vi "Spaceship_Draw.vi"(1 "Spaceship_data out":T1) -> (0 "SpaceshipLines":cluster{"x":i16, "y":i16}[](array[cluster]))   [LabVIEW 2017]
uses:
  Spaceship_data.ctl
  GameConfig/GameConfig_data.ctl
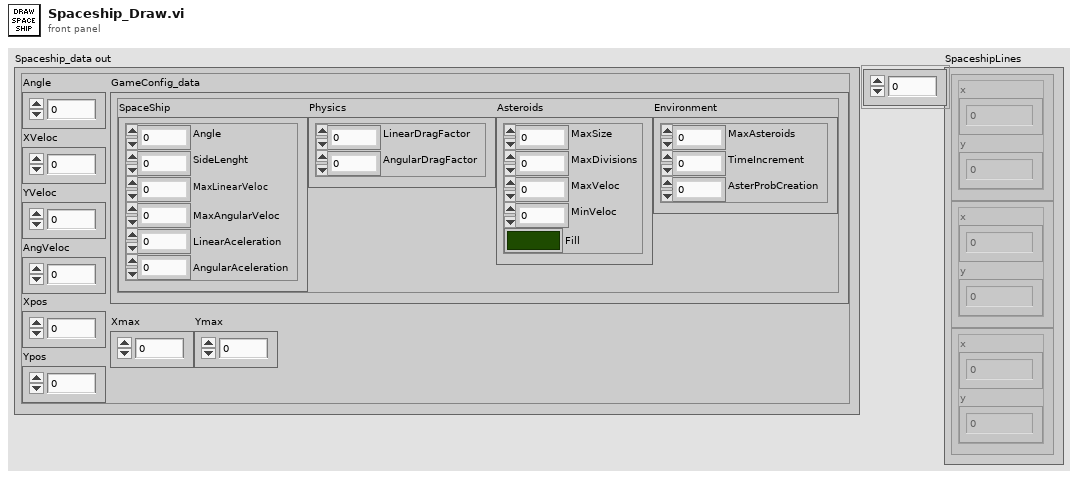
[diagram p1: front panel]
types:
  T1 = typedef "Spaceship_data.ctl" = cluster{"Angle":dbl, "XVeloc":dbl, "YVeloc":dbl, "AngVeloc":dbl, "GameConfig_data":T2, "Xpos":dbl, "Ypos":dbl, "Xmax":dbl, "Ymax":dbl}
  T2 = typedef "GameConfig_data.ctl" = cluster{"SpaceShip":cluster{"Angle":dbl, "SideLenght":dbl, "MaxLinearVeloc":dbl, "MaxAngularVeloc":dbl, "LinearAceleration":dbl, "AngularAceleration":dbl}, "Physics":cluster{"LinearDragFactor":dbl, "AngularDragFactor":dbl}, "Asteroids":cluster{"MaxSize":dbl, "MaxDivisions":i32, "MaxVeloc":dbl, "MinVeloc":dbl, "Fill":bool}, "Environment":cluster{"MaxAsteroids":i32, "TimeIncrement":dbl, "AsterProbCreation":dbl}}
  T3 = cluster{"Angle":dbl, "SideLenght":dbl, "MaxLinearVeloc":dbl, "MaxAngularVeloc":dbl, "LinearAceleration":dbl, "AngularAceleration":dbl}
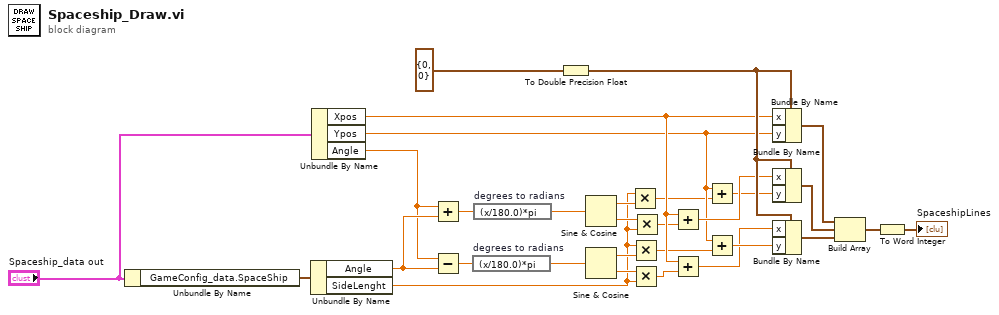
[diagram p0: block diagram]
diagram:
  n1 = Unbundle By Name("Spaceship_data out") -> ("GameConfig_data.SpaceShip"=w28:T3)
  n2 = Unbundle By Name(w28) -> ("Angle"=w27:dbl, "SideLenght"=w3:dbl)
  n3 = Unbundle By Name("Spaceship_data out") -> ("Xpos"=w20:dbl, "Ypos"=w19:dbl, "Angle"=w26:dbl)
  n4 = Add(x=w26, y=w27) -> (x+y=w11:dbl)
  n5 = Subtract(x=w26, y=w27) -> (x-y=w13:dbl)
  n6 = expression code="(x/180.0)*pi" "degrees to radians"(w13) -> (w12:dbl)
  n7 = expression code="(x/180.0)*pi" "degrees to radians"(w11) -> (w10:dbl)
  n8 = To Double Precision Float(number=cluster{"x":i16, "y":i16} {"x"=0, "y"=0}) -> (double precision float=w30:cluster{"x":dbl, "y":dbl})
  n9 = Sine & Cosine(0:w10) -> (1:w5:dbl, 2:w4:dbl)
  n10 = Sine & Cosine(0:w12) -> (1:w7:dbl, 2:w9:dbl)
  n11 = Multiply(x=w3, y=w5) -> (x*y=w1:dbl)
  n12 = Multiply(x=w3, y=w7) -> (x*y=w6:dbl)
  n13 = Multiply(x=w9, y=w3) -> (x*y=w8:dbl)
  n14 = Multiply(x=w4, y=w3) -> (x*y=w2:dbl)
  n15 = Add(x=w20, y=w2) -> (x+y=w24:dbl)
  n16 = Add(x=w20, y=w8) -> (x+y=w21:dbl)
  n17 = Add(x=w19, y=w1) -> (x+y=w23:dbl)
  n18 = Add(x=w19, y=w6) -> (x+y=w22:dbl)
  n19 = Bundle By Name(cluster=w30, "x"=w20, "y"=w19) -> (w16:cluster{"x":dbl, "y":dbl})
  n20 = Bundle By Name(cluster=w30, "x"=w24, "y"=w23) -> (w17:cluster{"x":dbl, "y":dbl})
  n21 = Bundle By Name(cluster=w30, "x"=w21, "y"=w22) -> (w18:cluster{"x":dbl, "y":dbl})
  n22 = Build Array(w16, w17, w18) -> (w15:cluster{"x":dbl, "y":dbl}[])
  n23 = To Word Integer(number=w15) -> (16bit integer=→"SpaceshipLines":cluster{"x":i16, "y":i16}[])
